vi "Read Node from VIPB.vi"(8 "error in (no error)":errorcluster, 10 "XPath expression":string, 11 "VIPB File Path":path) -> (0 "error out":errorcluster, 2 "node text":string, 3 "VIPB File Path out":path)   [LabVIEW 2019, in "VIPM.lvlib"]
uses:
  VIPM.lvlib
  <vilib>/xml/Close Reference(Node).vi
  <vilib>/xml/NI_XML.lvlib
  <resource>/objmgr/DOMUserDefRef.rc
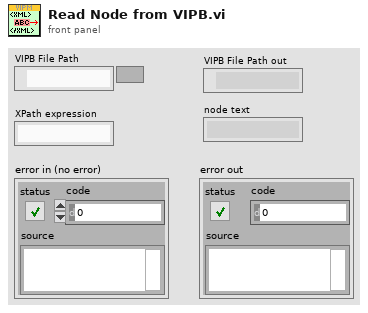
[diagram p1: front panel]
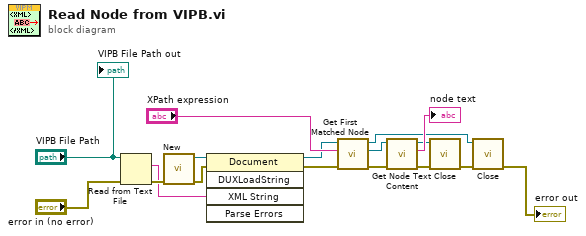
[diagram p0: block diagram]
diagram:
  n1 = Read from Text File(file (use dialog)="VIPB File Path", error in="error in (no error)") -> (text=w5:string, error out=w10:errorcluster)  [unwired: 2 in, 2 out]
  n2 = call <vilib>:"New.vi"("error in (no error)"=w10) -> ("error out"=w11:errorcluster, "DOM document out"=w4:refnum<k20>)  [unwired: 7 in]
  n3 = invoke class="Document" method="DUXLoadString"(reference=w4, error in=w11, "XML String"=w5) -> (reference out=w2:refnum<k20>, error out=w1:errorcluster)  [unwired: 2 in, 3 out]
  n4 = call <vilib>:"Get First Matched Node.vi"("error in (no error)"=w1, "XPath expression"="XPath expression", "node in"=w2) -> ("error out"=w12:errorcluster, "node result"=w7:refnum<k20>, "node out"=w6:refnum<k20>)  [unwired: 6 in]
  n5 = call <vilib>:"Get Node Text Content.vi"("error in (no error)"=w12, "node in"=w7) -> ("error out"=w13:errorcluster, "node text"=→"node text":string, "node out"=w8:refnum<k20>)  [unwired: 7 in]
  n6 = call-poly <vilib>:"Close.vi"("error in (no error)"=w13, "node"=w8) -> ("error out"=w14:errorcluster)  [unwired: 7 in]
  n7 = call-poly <vilib>:"Close.vi"("error in (no error)"=w14, "node"=w6) -> ("error out"=→"error out":errorcluster)  [unwired: 7 in]
  "VIPB File Path out" <- "VIPB File Path"
